vi "PMJD T027 SubVI04.vi"(1 "Q":dbl, 2 "P":dbl, 3 "f":dbl[][](array[numeric])) -> (0 "mpq":dbl)   [LabVIEW 2020]
doc: "PINEDA MENDEZ JOB DANIEL 4MV6 SVA 2022/1\nT027 SubVI04\nEste subvi calcula los momentos iniciales (mpq) dados los parametros P, Q y f"
panel:
  # "PINEDA MENDEZ JOB DANIEL    4MV6    SVA    2022/1\nT027     SubVI04    Calculo de momentos iniciales mpq"
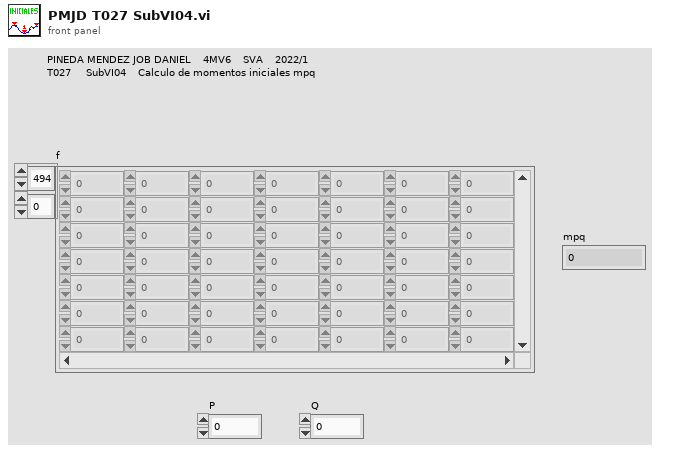
[diagram p1: front panel]
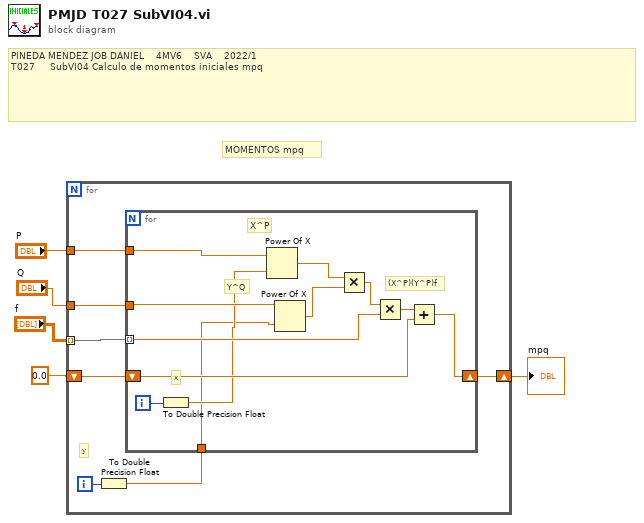
[diagram p0: block diagram]
diagram:
  # "PINEDA MENDEZ JOB DANIEL    4MV6    SVA    2022/1\nT027     SubVI04 Calculo de momentos iniciales mpq"
  # "MOMENTOS mpq"
  n1 = for {
    tunnel: "f" -> [w12] mode=indexing
    tunnel: "P" -> [w11]
    tunnel: "Q" -> [w10]
    shift-right: [w9] -> w1
    shift-left: 0.0 -> [w8]
    i -> [w7]
    # "y"
    n2 = To Double Precision Float(number=w7) -> (double precision float=w6:dbl)
    n3 = for {
      tunnel: w12 -> [w15] mode=indexing
      tunnel: w11 -> [w24]
      tunnel: w10 -> [w22]
      shift-right: [w17] -> w9
      shift-left: w8 -> [w16]
      tunnel: w6 -> [w13]
      i -> [w23]
      # "x"
      # "(X^P)(Y^P)f"
      # "Y^Q"
      # "X^P"
      n4 = To Double Precision Float(number=w23) -> (double precision float=w14:dbl)
      n5 = Power Of X(1:w14, 2:w24) -> (0:w21:dbl)
      n6 = Power Of X(1:w13, 2:w22) -> (0:w20:dbl)
      n7 = Multiply(x=w21, y=w20) -> (x*y=w19:dbl)
      n8 = Multiply(x=w19, y=w15) -> (x*y=w18:dbl)
      n9 = Add(x=w18, y=w16) -> (x+y=w17:dbl)
    }
  }
  "mpq" <- w1
